vi "Greenhouse.vi"() -> ()   [LabVIEW 2020]
uses:
  <vilib>/Instr/_visa.llb/VISA Configure Serial Port (Instr).vi
panel:
  out "Personal":bool
  out "Thermometer":dbl(slide) scale=0.0..60.0
  out "hambiente":dbl(knob) scale=0.0..100.0
  out "Boolean":bool
  out "Tank":dbl(slide) scale=0.0..1000.0
  out "htierra":dbl(knob) scale=0.0..1000.0
  in  "stop":bool
  in  "VISA resource name":refnum<visa-resource-name>
  # "SISTEMA DE MONITOREO INVERNADERO"
  # "SELECCIÓN SERIAL"
  # "MONITOREO DE TIERRA"
  # "RPM"
  # "HUMEDAD"
  # "NIVEL DEL TANQUE"
  # "ACTIVAR \nLLENADO"
  # "MONITOREO DE AMBIENTE"
  # "HUMEDAD"
  # "TEMPERATURA"
  # "PERSONAL"
  # "PERSONAL\nTRABAJANDO"
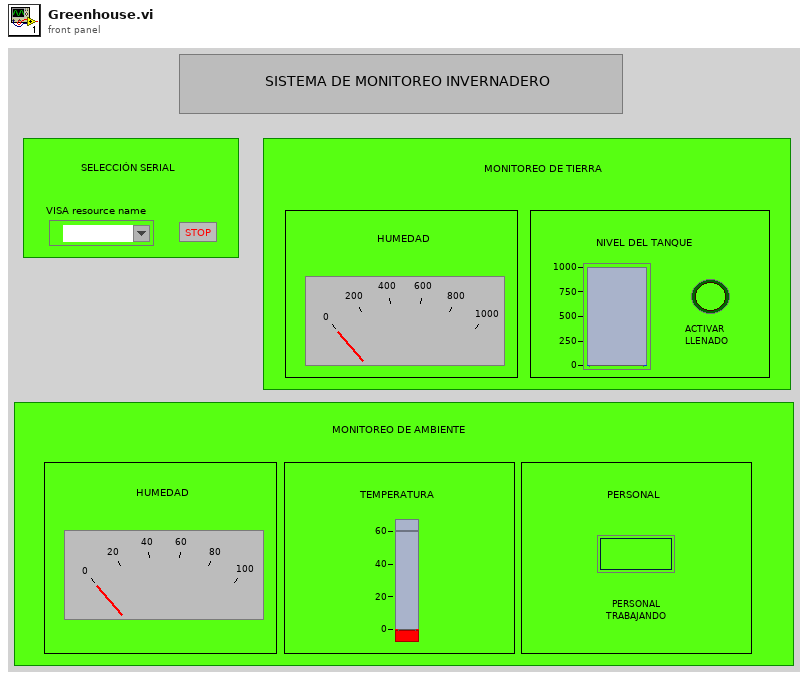
[diagram p1: front panel]
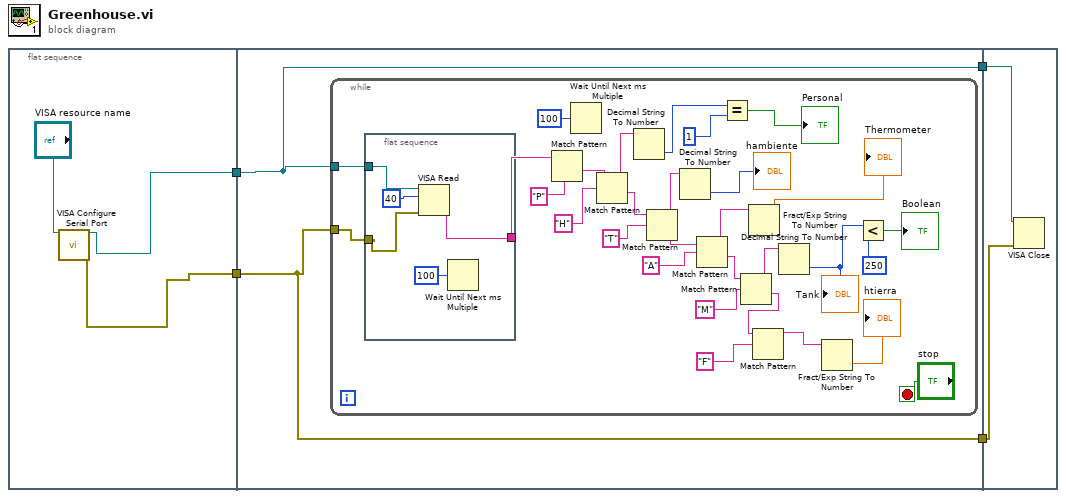
[diagram p0: block diagram]
diagram:
  n1 = flat-sequence {
    tunnel: [w6] -> w4
    tunnel: [w5] -> w3
    tunnel: w4 -> [w9]
    tunnel: w3 -> [w8]
    tunnel: [w9] -> w2
    tunnel: [w8] -> w1
    tunnel: w2 -> [w46]
    tunnel: w1 -> [w45]
    frame #0 {
      n2 = call-poly "VISA Configure Serial Port"("VISA resource name"="VISA resource name") -> ("VISA resource name out"=w6:refnum<visa-resource-name>, "error out"=w5:errorcluster)  [unwired: 13 in]
    }
    frame #1 {
      n3 = while {
        tunnel: w8 -> [w39]
        tunnel: w9 -> [w26]
        stop <- "stop" stop-if-true
        n4 = flat-sequence {
          tunnel: w26 -> [w44]
          tunnel: w39 -> [w43]
          tunnel: [w42] -> w38
          frame #0 {
            n5 = VISA Read(VISA resource name=w44, byte count=u32 40, error in (no error)=w43) -> (read buffer=w42:string)  [unwired: 3 out]
            n6 = Wait Until Next ms Multiple(millisecond multiple=u32 100) -> ()  [unwired: 1 out]
          }
        }
        n7 = Match Pattern(string=w38, regular expression="P") -> (after substring=w35:string)  [unwired: 1 in, 3 out]
        n8 = Wait Until Next ms Multiple(millisecond multiple=u32 100) -> ()  [unwired: 1 out]
        n9 = Match Pattern(string=w35, regular expression="H") -> (before substring=w34:string, after substring=w30:string)  [unwired: 1 in, 2 out]
        n10 = Decimal String To Number(string=w34) -> (number=w25:i32)  [unwired: 2 in, 1 out]
        n11 = Match Pattern(string=w30, regular expression="T") -> (before substring=w29:string, after substring=w31:string)  [unwired: 1 in, 2 out]
        n12 = Decimal String To Number(string=w29) -> (number=→"hambiente":i32)  [unwired: 2 in, 1 out]
        n13 = Match Pattern(string=w31, regular expression="A") -> (before substring=w13:string, after substring=w21:string)  [unwired: 1 in, 2 out]
        n14 = Equal?(x=w25, y=1) -> (x = y?=→"Personal":bool)
        n15 = Match Pattern(string=w21, regular expression="M") -> (before substring=w19:string, after substring=w18:string)  [unwired: 1 in, 2 out]
        n16 = Fract/Exp String To Number(string=w13) -> (number=→"Thermometer":dbl)  [unwired: 3 in, 1 out]
        n17 = Match Pattern(string=w18, regular expression="F") -> (before substring=w11:string)  [unwired: 1 in, 3 out]
        n18 = Decimal String To Number(string=w19) -> (number=w15:i32)  [unwired: 2 in, 1 out]
        "Tank" <- w15
        n19 = Fract/Exp String To Number(string=w11) -> (number=→"htierra":dbl)  [unwired: 3 in, 1 out]
        n20 = Less?(x=w15, y=250) -> (x < y?=→"Boolean":bool)
      }
    }
    frame #2 {
      n21 = VISA Close(VISA resource name=w46, error in (no error)=w45) -> ()  [unwired: 1 out]
    }
  }
